vi "TEST - Variant Constant.vi"(8 "error in (no error)":errorcluster) -> (0 "error out":errorcluster, 2 "Pass":bool)   [LabVIEW 2020]
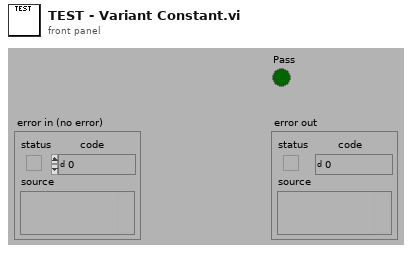
[diagram p1: front panel]
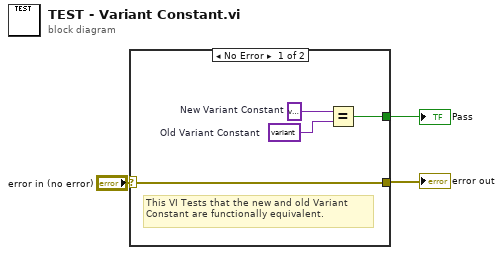
[diagram p0: block diagram]
diagram:
  n1 = case shown="No Error" "error in (no error)" {
    selector: "error in (no error)" -> [w7 w8]
    tunnel: [w4 _] -> w3
    tunnel: [w7 w8] -> w1
    frame No Error {
      w5 = variant  # New Variant Constant
      w6 = variant  # Old Variant Constant
      # "This VI Tests that the new and old Variant Constant are functionally equivalent."
      n2 = Equal?(x=w5, y=w6) -> (x = y?=w4:bool)
    }
    frame Error {
    }
  }
  "Pass" <- w3
  "error out" <- w1
